vi "getTags.vi"(8 "error in (no error)":errorcluster, 11 "IComponent in":refnum<class "IComponent.lvclass">) -> (0 "error out":errorcluster, 3 "IComponent out":refnum<class "IComponent.lvclass">)   [LabVIEW 2022 SP3, in "openDAQ.lvlib" / "IBaseObject.lvlib" / "IPropertyObject.lvlib" / "IComponent.lvlib" / "IComponent.lvclass"]
uses:
  <instrlib>/openDAQ/Public/Classes/IComponent/IComponent.lvclass
  <instrlib>/openDAQ/Public/Classes/IComponent/IComponent.lvclass/IComponent.ctl
  <instrlib>/openDAQ/Public/Classes/ITags/ITags.lvclass
  <instrlib>/openDAQ/Binaries/Windows/x86/copendaq32.dll
panel:
  out "ITags out":refnum<class "ITags.lvclass">
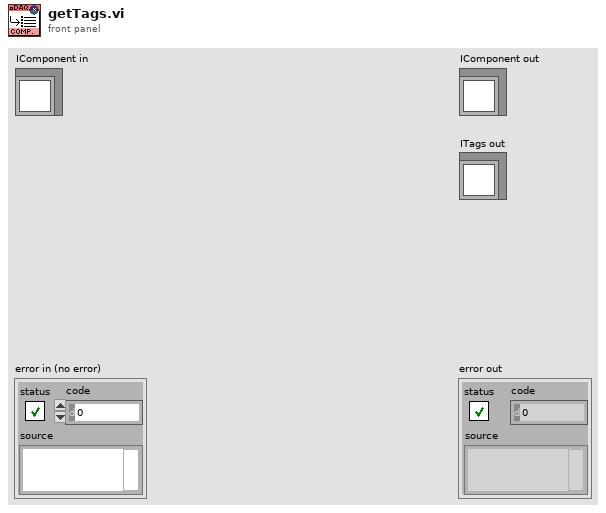
[diagram p1: front panel]
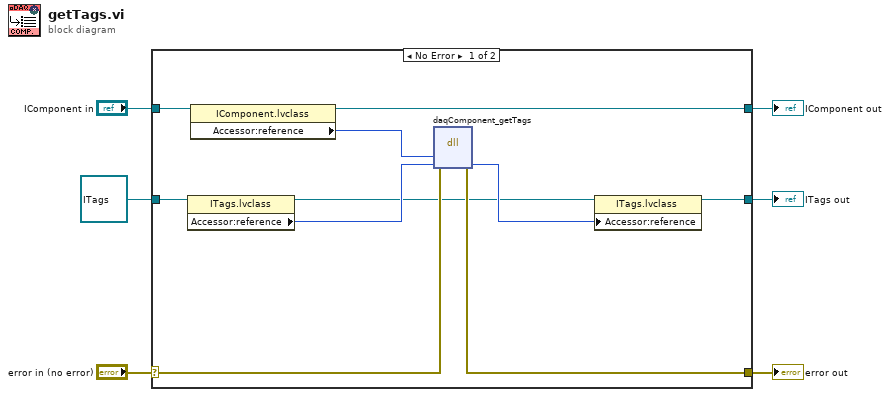
[diagram p0: block diagram]
diagram:
  n1 = case shown="No Error" "error in (no error)" {
    selector: "error in (no error)" -> [w11 w19]
    tunnel: [w14 w19] -> w5
    tunnel: [w12 w18] -> w3
    tunnel: "IComponent in" -> [w13 w18]
    tunnel: [w8 w17] -> w1
    tunnel: refnum<class "ITags.lvclass"> refnum ("openDAQ.lvlib:IBaseObject.lvlib:ITag.lvlib:ITag.lvclass") -> [w7 w17]
    frame No Error {
      n2 = property class="ITags.lvclass"(reference=w7) -> (reference out=w10:refnum<class "ITags.lvclass">, "Accessor:reference"=w15:i64)  [unwired: 1 in, 1 out]
      n3 = property class="IComponent.lvclass"(reference=w13) -> (reference out=w12:refnum<class "IComponent.lvclass">, "Accessor:reference"=w9:i64)  [unwired: 1 in, 1 out]
      n4 = dll-call lib="C:/Program Files (x86)/National Instruments/LabVIEW 2022/instr.lib/openDAQ/Binaries/Windows/x86/copendaq*.*" fn="daqComponent_getTags"(error in=w11, "component"=w9, "tags"=w15) -> (error out=w14:errorcluster, "tags"=w16:i64)  [unwired: 4 in, 1 out]
      n5 = property class="ITags.lvclass"(reference=w10, "Accessor:reference"=w16) -> (reference out=w8:refnum<class "ITags.lvclass">)  [unwired: 1 in, 1 out]
    }
    frame Error {
    }
  }
  "error out" <- w5
  "IComponent out" <- w3
  "ITags out" <- w1
